vi "String.Float to String, No Trailing Zeros.vi"(11 "Numeric":dbl) -> (3 "String":string)   [LabVIEW 2024, in "EQMF.lvlib" / "String Utils.lvlib"]
uses:
  String Utils.lvlib
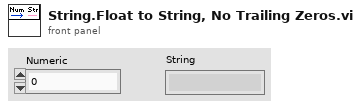
[diagram p1: front panel]
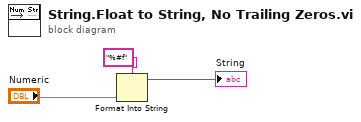
[diagram p0: block diagram]
diagram:
  n1 = Format Into String(format string="%#f", "Numeric") -> (resulting string=→"String":string)  [unwired: 2 in, 1 out]
